vi "DSF.Shared.Configuration.Transfer.Find First Instance.vi"(8 "error in (no error)":errorcluster, 11 "objects":refnum<class>[](array[class])) -> (0 "error out":errorcluster, 2 "found?":bool, 3 "Transfer Configuration":refnum<class "DSF.Shared.Configuration.Transfer.lvclass">)   [LabVIEW 2016, in "DSF.Shared.lvlib" / "DSF.Shared.Configuration.Transfer.lvclass"]
uses:
  DSF.Shared.Configuration.Transfer.lvclass
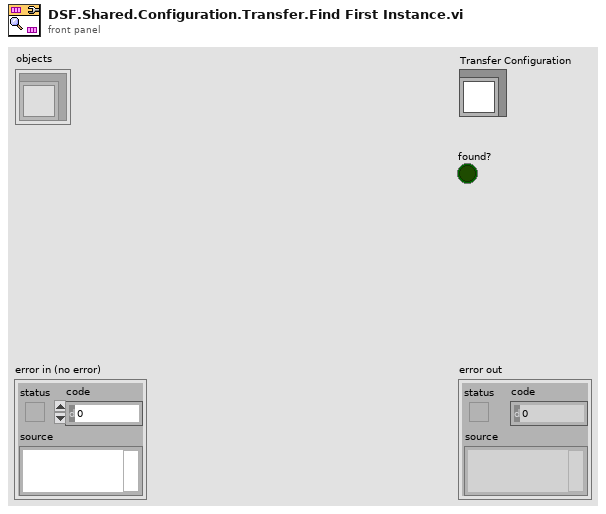
[diagram p1: front panel]
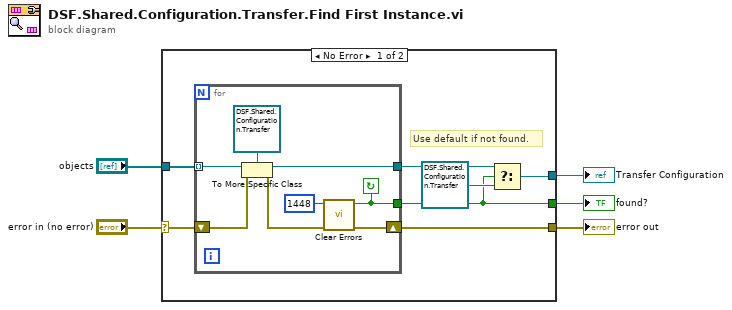
[diagram p0: block diagram]
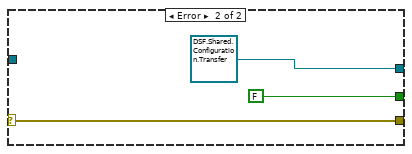
[diagram p2: hidden frame]
diagram:
  n1 = case shown="No Error" "error in (no error)" {
    selector: "error in (no error)" -> [w11 w23]
    tunnel: "objects" -> [w12 _]
    tunnel: [w10 w23] -> w1
    tunnel: [w8 refnum<class "DSF.Shared.Configuration.Transfer.lvclass"> refnum ("Transfer Configuration in")] -> w4
    tunnel: [w6 FALSE ("specific error cleared?")] -> w3
    frame No Error {
      # "Use default if not found."
      n2 = for {
        tunnel: w12 -> [w19] mode=indexing
        tunnel: [w18] -> w9
        shift-right: [w14] -> w10
        shift-left: w11 -> [w16]
        tunnel: [w13] -> w6
        stop <- w13 continue-if-true
        n3 = To More Specific Class(target class=refnum<class "DSF.Shared.Configuration.Transfer.lvclass"> refnum ("Transfer Configuration in"), reference=w19, error in=w16) -> (specific class reference=w18:refnum<class "DSF.Shared.Configuration.Transfer.lvclass">, error out=w15:errorcluster)
        n4 = call <vilib>:"Clear Errors.vi"("error in (no error)"=w15, "specific error code to clear (0: all)"=1448) -> ("error out"=w14:errorcluster, "specific error cleared?"=w13:bool)  [unwired: 4 in]
      }
      n5 = Select(t=w9, s=w6, f=refnum<class "DSF.Shared.Configuration.Transfer.lvclass"> refnum) -> (s? t:f=w8:refnum<class "DSF.Shared.Configuration.Transfer.lvclass">)
    }
    frame Error {
    }
  }
  "error out" <- w1
  "Transfer Configuration" <- w4
  "found?" <- w3
